vi "IRC-Clip-Ball_Api.vi"(8 "Error In":errorcluster, 11 "目標電壓":dbl[](array[numeric])=[0.0, 0.0, 0.0, 0.0, 0.0, 0.0, 0.0, 1.48777]) -> (0 "Error Out":errorcluster)   [LabVIEW 2019]
uses:
  <vilib>/Platform/TimedLoop/XDataNode/timing_clust.ctl
  <vilib>/Platform/TimedLoop/XDataNode/nitl_modes.ctl
  <vilib>/Platform/TimedLoop/XDataNode/wakeup.ctl
  <vilib>/platform/TimedLoop/XDataNode/XDataNode.xnode
  <vilib>/Platform/TimedLoop/XDataNode/XDNodeRunTimeDep.lvlib
panel:
  in  "Stop":bool
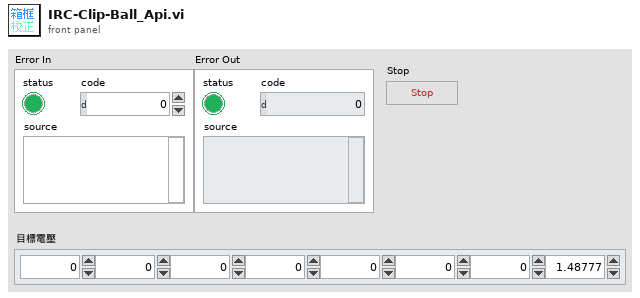
[diagram p1: front panel]
types:
  T1 = typedef "XDNodeRunTimeDep.lvlib/timing_clust.ctl" = cluster{"Expected End [f-1]":u64, "Actual End [f-1]":u64, "Finished Late? [f-1]":bool, "Expected End [i-1]":u64, "Actual End [i-1]":u64, "Finished Late? [i-1]":bool, "Expected Start [i]":u64, "Actual Start [i]":u64, "Expected Start [f]":u64, "Actual Start [f]":u64, "Source Name":string, "Structure Name":string, "Period":i64, "Deadline":i64, "Offset":i64, "Start":i64, "Priority":i32, "Timeout":i32, "Mode":T2, "Wakeup Reason":T3, "Error":errorcluster, "Source Type":string, "Secondary Source Type":string, "Global End Time":u64, "Global Start Time":u64, "Frame Duration":u64, "Iteration Duration":u64, "Assigned CPU":i32, "I/O Scan Engine Mode":u32}
  T2 = typedef "XDNodeRunTimeDep.lvlib/nitl_modes.ctl" = enum32{"No Change", "Process missed periods, maintain original phase", "Discard missed periods, maintain original phase", "Process missed periods, ignore original phase", "Discard missed periods, ignore original phase"}
  T3 = typedef "XDNodeRunTimeDep.lvlib/wakeup.ctl" = enum32{"Normal", "Aborted", "Asynchronous wakeup", "Timing source error", "Timed loop error", "Timeout"}
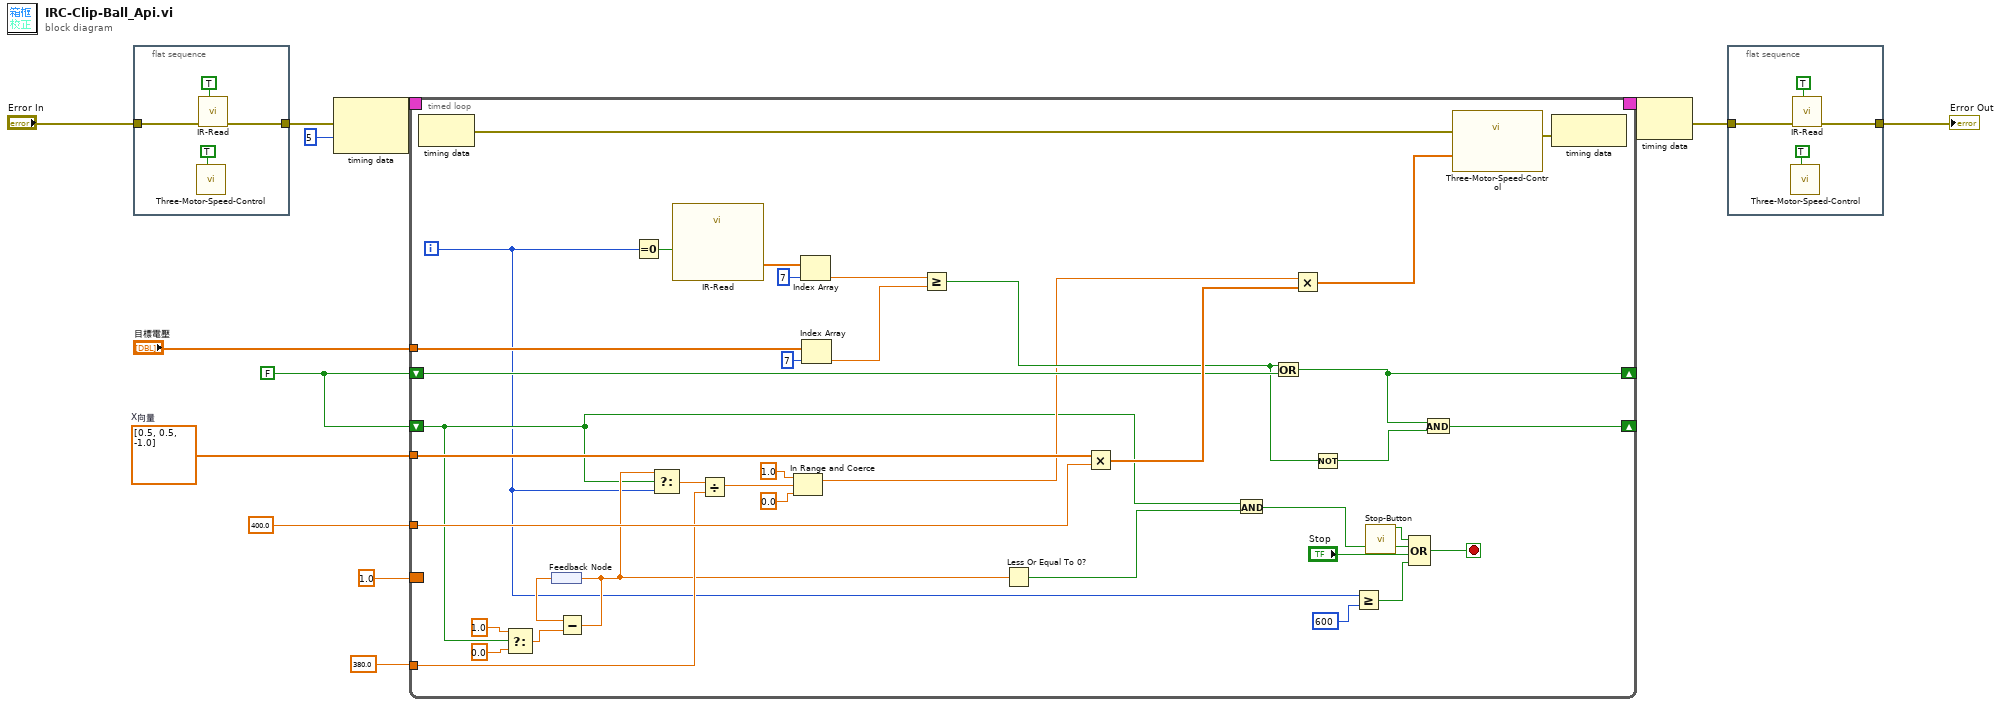
[diagram p0: block diagram]
diagram:
  w7 = FALSE
  w9 = dbl[] [0.5, 0.5, -1.0]  # X向量
  n1 = flat-sequence {
    tunnel: "Error In" -> [w17]
    tunnel: [w16] -> w5
    frame #0 {
      n2 = call "Three-Motor-Speed-Control.vi"("Reset"=TRUE) -> ()  [unwired: 10 in, 1 out]
      n3 = call "IR-Read.vi"("Reset"=TRUE, "Error In"=w17) -> ("Error Out"=w16:errorcluster)  [unwired: 8 in, 1 out]
    }
  }
  n4 = node-c288(w5, i64 5 ("Period")) -> (w13:T1)
  n5 = timed-loop {
    timing: w13 -> [_]
    timing-out: [_] -> w12
    tunnel: "目標電壓" -> [w49]
    tunnel: w9 -> [w40]
    tunnel: 400.0 -> [w39]
    shift-right: [w21] -> _
    shift-left: w7 -> [w36]
    shift-right: [w33] -> _
    shift-left: w7 -> [w24]
    border: 1.0 -> [_]
    tunnel: 380.0 -> [w29]
    i -> [w19]
    stop <- w55 stop-if-true
    n6 = node-c288() -> (w52:errorcluster)  [unwired: 1 in]
    n7 = Select(t=1.0, s=w24, f=0.0) -> (s? t:f=w28:dbl)
    n8 = feedback #1() -> (w32:dbl)
    n9 = Subtract(x=w32, y=w28) -> (x-y=w25:dbl)
    n10 = feedback-in #1(w25) -> ()
    n11 = Equal To 0?(x=w19) -> (x = 0?=w51:bool)
    n12 = Select(t=w25, s=w24, f=w19) -> (s? t:f=w30:dbl)
    n13 = call "IR-Read.vi"("Reset"=w51) -> ("輸出紅外線值"=w50:dbl[])  [unwired: 9 in, 1 out]
    n14 = Divide(x=w30, y=w29) -> (x/y=w44:dbl)
    n15 = In Range and Coerce(upper limit=1.0, x=w44, lower limit=0.0) -> (coerced(x)=w31:dbl)  [unwired: 1 out]
    n16 = Index Array(array=w50, index=7) -> (element=w46:dbl)
    n17 = Index Array(array=w49, index=7) -> (element=w47:dbl)
    n18 = Greater Or Equal?(x=w46, y=w47) -> (x >= y?=w34:bool)
    n19 = Less Or Equal To 0?(x=w25) -> (x <= 0?=w23:bool)
    n20 = Multiply(x=w40, y=w39) -> (x*y=w41:dbl[])
    n21 = And(x=w24, y=w23) -> (x .and. y?=w22:bool)
    n22 = Or(x=w34, y=w36) -> (x .or. y?=w21:bool)
    n23 = Multiply(x=w31, y=w41) -> (x*y=w38:dbl[])
    n24 = Not(x=w34) -> (.not. x?=w35:bool)
    n25 = Greater Or Equal?(x=w19, y=600) -> (x >= y?=w20:bool)
    n26 = call "Stop-Button.vi"() -> ("顯示按下?"=w45:bool)  [unwired: 10 in, 1 out]
    n27 = Compound Arithmetic op=OR(w45, w22, "Stop", w20) -> (w55:bool)
    n28 = And(x=w21, y=w35) -> (x .and. y?=w33:bool)
    n29 = call "Three-Motor-Speed-Control.vi"("Error In"=w52, "速度(秒/度)"=w38) -> ("Error Out"=w53:errorcluster)  [unwired: 9 in]
    n30 = node-c288(w53) -> ()  [unwired: 1 out]
  }
  n31 = node-c288(w12) -> (w4:errorcluster)
  n32 = flat-sequence {
    tunnel: w4 -> [w64]
    tunnel: [w63] -> w3
    frame #0 {
      n33 = call "Three-Motor-Speed-Control.vi"("Reset"=TRUE) -> ()  [unwired: 10 in, 1 out]
      n34 = call "IR-Read.vi"("Reset"=TRUE, "Error In"=w64) -> ("Error Out"=w63:errorcluster)  [unwired: 8 in, 1 out]
    }
  }
  "Error Out" <- w3
